vi "Subvi counter U64.vi"(8 "Reset":bool, 9 "+1":bool) -> (1 "Output":u64)   [LabVIEW 2017]
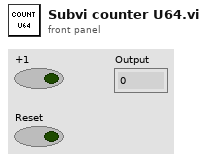
[diagram p1: front panel]
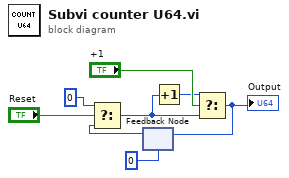
[diagram p0: block diagram]
diagram:
  n1 = feedback #1(u64 0) -> (w6:u64)
  n2 = Select(t=u64 0, s="Reset", f=w6) -> (s? t:f=w5:u64)
  n3 = Increment(x=w5) -> (x+1=w1:u64)
  n4 = Select(t=w1, s="+1", f=w5) -> (s? t:f=w3:u64)
  "Output" <- w3
  n5 = feedback-in #1(w3) -> ()
